vi "Save Settings to XML.vi"(8 "error in (no error)":errorcluster, 11 "Settings":T1={"Acq Settings"={"Instrument Specifications"=[], "Config Settings"={"Simulated Sensor Injection"=0.0, "Base Device Name"="", "Simulation Mode"=""}}, "Processing Settings"={"Sensor CoreData"=[], "Test Parameters"=[], "Measurement Roles"=[], "Test Sequence Context"=[]}, "Session Identifiers"={"SerialNumber"=[], "OperatorName"=""}, "Test Sequence Settings"={"Test Sequence State"={"Test Sequence Enum"=enum."Idle", "Point Index"=0, "Current Target"=0.0, "Previous Target"=0.0, "Simulation?"=TRUE, "Direction"=enum."Acsending", "Transition Active?"=FALSE, "Cycle Number"=0}}, "Stimulus Settings"={"Stimulus Outputs"=[]}} {"Processing Settings"."Test Parameters"."Allowed Tolerance (%) FS" format="%#_4g"; "Acq Settings"."Config Settings"."Simulated Sensor Injection" scale=0.0..100.0}) -> (0 "error out":errorcluster)   [LabVIEW 2026, in "Settings.lvlib"]
doc: "Saves the \"User Specified\" configuration data to an XML file. This is used to remember the users settings between executions."
uses:
  Settings.lvlib
  <vilib>/Utility/xml.llb/Write to XML File(string).vi
  Acquisition/Instrument Specifications Configuration.ctl
  Acquisition/Acquisition.lvlib
  controls/UI/Settings Cluster.ctl
  controls/UI/Measurement Role.ctl
  Acquisition/Instrument Specifications Cluster Configuration.ctl
  controls/UI/Config Settings.ctl
  controls/UI/Acq Settings.ctl
  controls/UI/Units Enum.ctl
  controls/UI/Signal Enum.ctl
  controls/Messaging Payloads/Sensor CoreData Cluster.ctl
  controls/Messaging Payloads/Sensor CoreData.ctl
  Processing/Test Parameters Cluster.ctl
  Processing/Test Parameters.ctl
  Processing/Processing_Engine.lvlib
  controls/UI/Direction.ctl
  controls/UI/Test Sequence Context Cluster.ctl
  controls/UI/Test Sequence Context.ctl
  Processing/Processing Settings.ctl
  controls/UI/Session Identfiers.ctl
  controls/UI/Test Sequence Enum.ctl
  controls/UI/Test Sequence State.ctl
  controls/UI/Test Sequence Settings.ctl
  controls/Controller/Controller Core Data.ctl
  controls/Controller/Stimulus Role.ctl
  controls/Controller/Stimulus Output Configuration.ctl
  controls/Controller/Stimulus Output.ctl
  controls/Controller/Stimulus Outputs.ctl
  controls/Controller/Stimulus Settings.ctl
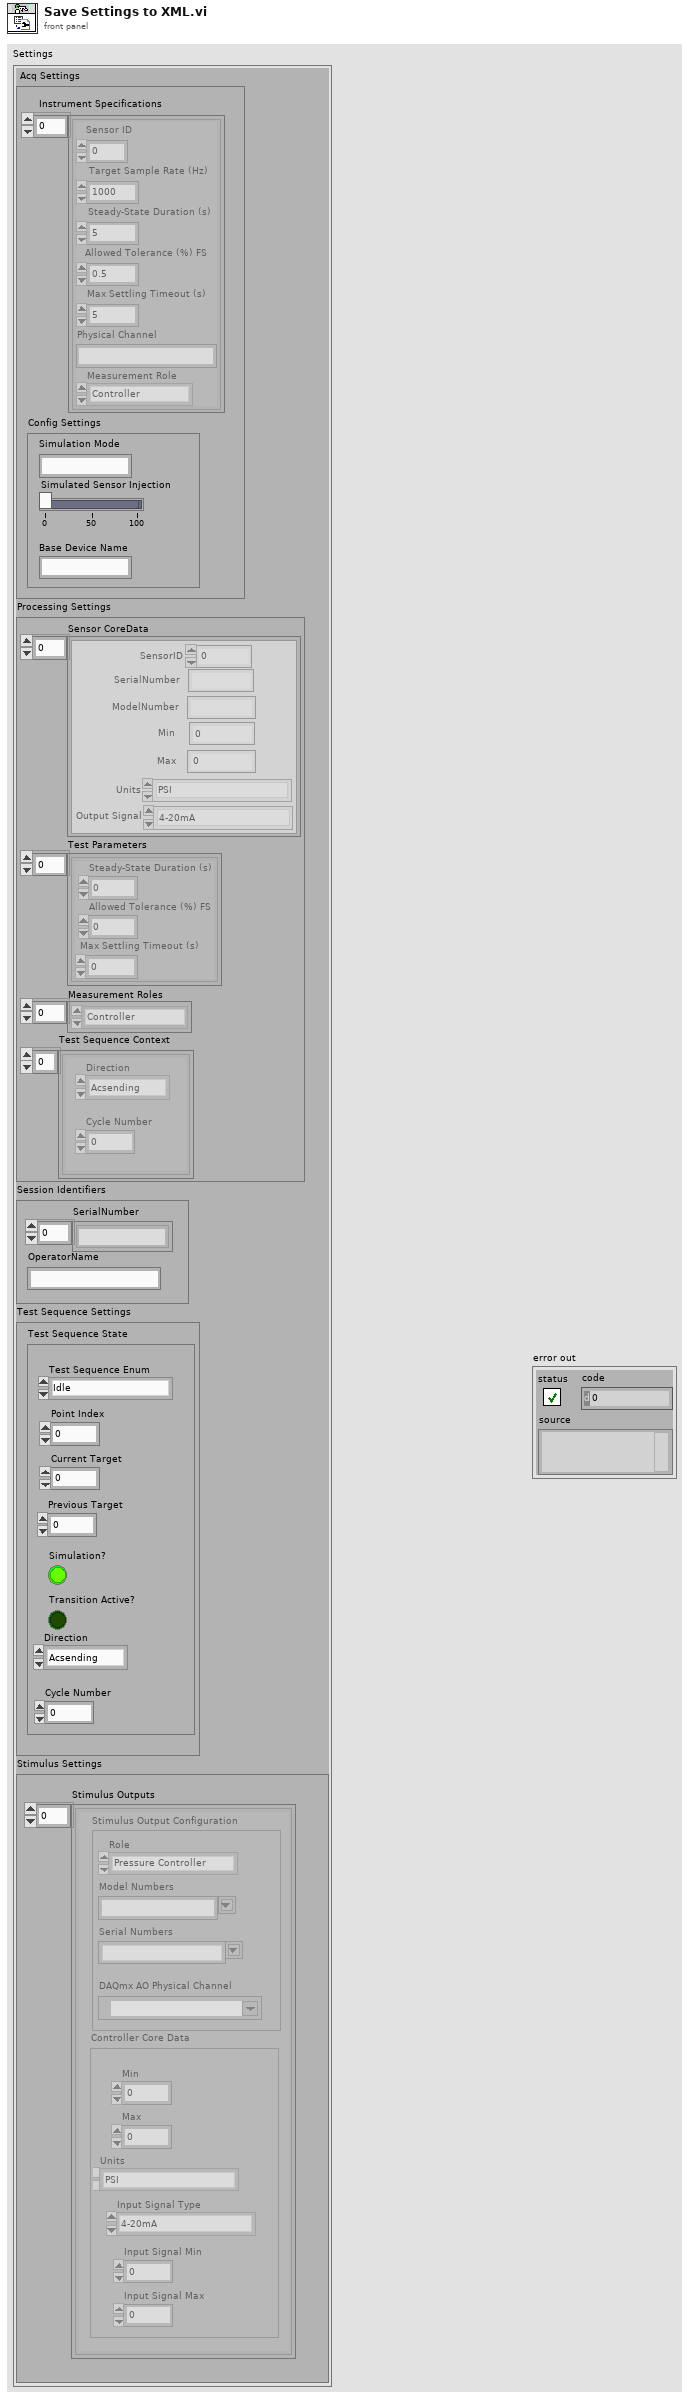
[diagram p1: front panel]
types:
  T1 = typedef "Settings Cluster.ctl" = cluster{"Acq Settings":T2, "Processing Settings":T7, "Session Identifiers":T17, "Test Sequence Settings":T18, "Stimulus Settings":T21}
  T2 = typedef "Acq Settings.ctl" = cluster{"Instrument Specifications":T3, "Config Settings":T6}
  T3 = typedef "Acquisition.lvlib/Instrument Specifications Configuration.ctl" = T4[]
  T4 = typedef "Acquisition.lvlib/Instrument Specifications Cluster Configuration.ctl" = cluster{"Sensor ID":i32, "Target Sample Rate (Hz)":dbl, "Steady-State Duration (s)":i32, "Allowed Tolerance (%) FS":dbl, "Max Settling Timeout (s)":i32, "Physical Channel":string, "Measurement Role":T5}
  T5 = typedef "Settings.lvlib/Measurement Role.ctl" = enum16{"Controller", "Reference", "UUT", "Disable", "All"}
  T6 = typedef "Config Settings.ctl" = cluster{"Simulated Sensor Injection":dbl, "Base Device Name":string, "Simulation Mode":string}
  T7 = typedef "Processing_Engine.lvlib/Processing Settings.ctl" = cluster{"Sensor CoreData":T8, "Test Parameters":T12, "Measurement Roles":T5[], "Test Sequence Context":T14}
  T8 = typedef "Sensor CoreData.ctl" = T9[]
  T9 = typedef "Settings.lvlib/Sensor CoreData Cluster.ctl" = cluster{"SerialNumber":string, "ModelNumber":string, "Min":dbl, "Max":dbl, "Units":T10, "Output Signal":T11, "SensorID":i32}
  T10 = typedef "Units Enum.ctl" = enum16{"PSI", "Deg C", "kPa", "GPM"}
  T11 = typedef "Signal Enum.ctl" = enum16{"4-20mA", "0-10V", "Thermocouple Type K"}
  T12 = typedef "Processing_Engine.lvlib/Test Parameters.ctl" = T13[]
  T13 = typedef "Settings.lvlib/Test Parameters Cluster.ctl" = cluster{"Steady-State Duration (s)":i32, "Allowed Tolerance (%) FS":dbl, "Max Settling Timeout (s)":i32}
  T14 = typedef "Settings.lvlib/Test Sequence Context.ctl" = T15[]
  T15 = typedef "Settings.lvlib/Test Sequence Context Cluster.ctl" = cluster{"Direction":T16, "Cycle Number":i32}
  T16 = typedef "Settings.lvlib/Direction.ctl" = enum16{"Acsending", "Descending"}
  T17 = typedef "Session Identfiers.ctl" = cluster{"SerialNumber":string[], "OperatorName":string}
  T18 = typedef "Test Sequence Settings.ctl" = cluster{"Test Sequence State":T19}
  T19 = typedef "Settings.lvlib/Test Sequence State.ctl" = cluster{"Test Sequence Enum":T20, "Point Index":i32, "Current Target":dbl, "Previous Target":dbl, "Simulation?":bool, "Direction":T16, "Transition Active?":bool, "Cycle Number":i32}
  T20 = typedef "Test Sequence Enum.ctl" = enum16{"Idle", "Start Point", "Point Complete", "Test Complete", "Abort Test", "Reset"}
  T21 = typedef "Settings.lvlib/Stimulus Settings.ctl" = cluster{"Stimulus Outputs":T22}
  T22 = typedef "Settings.lvlib/Stimulus Outputs.ctl" = T23[]
  T23 = typedef "Settings.lvlib/Stimulus Output.ctl" = cluster{"Controller Core Data":T24, "Stimulus Output Configuration":T25}
  T24 = typedef "Settings.lvlib/Controller Core Data.ctl" = cluster{"Min":dbl, "Max":dbl, "Units":T10, "Input Signal Type":T11, "Input Signal Min":dbl, "Input Signal Max":dbl}
  T25 = typedef "Settings.lvlib/Stimulus Output Configuration.ctl" = cluster{"DAQmx AO Physical Channel":tag, "Role":T26, "Model Numbers":string, "Serial Numbers":string}
  T26 = typedef "Stimulus Role.ctl" = enum16{"Pressure Controller", "Temperature Controller"}
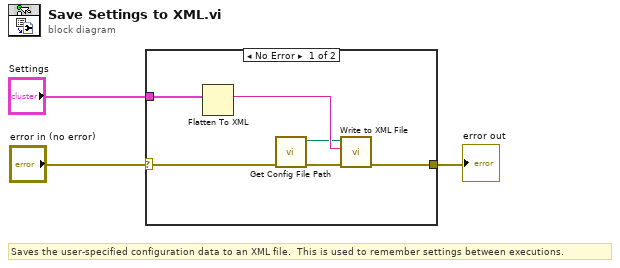
[diagram p0: block diagram]
diagram:
  # "Saves the user-specified configuration data to an XML file.  This is used to remember settings between executions."
  n1 = case shown="No Error" "error in (no error)" {
    selector: "error in (no error)" -> [w5 w10]
    tunnel: [w7 w10] -> w2
    tunnel: "Settings" -> [w9 _]
    frame No Error {
      n2 = Flatten To XML(6:w9) -> (2:w8:string)
      n3 = call "Get Config File Path.vi"("error in (no error)"=w5) -> ("error out"=w4:errorcluster, "XML File Path"=w6:path)  [unwired: 9 in]
      n4 = call-poly <vilib>:"Write to XML File.vi"("error in (no error)"=w4, "XML Input"=w8, "XML File Path"=w6) -> ("error out"=w7:errorcluster)  [unwired: 6 in, 2 out]
    }
    frame Error {
    }
  }
  "error out" <- w2
